vi "ASI_bufferToImage_Array.vi"(0 "iWidth":i32, 5 "iHeight":i32, 9 "imageType":i32, 11 "pBuffer in":u8[](array[numeric])) -> (10 "output array":u32[][](array[numeric]))   [LabVIEW 2023]
panel:
  in  "16bit type 2":u16[](array[numeric])
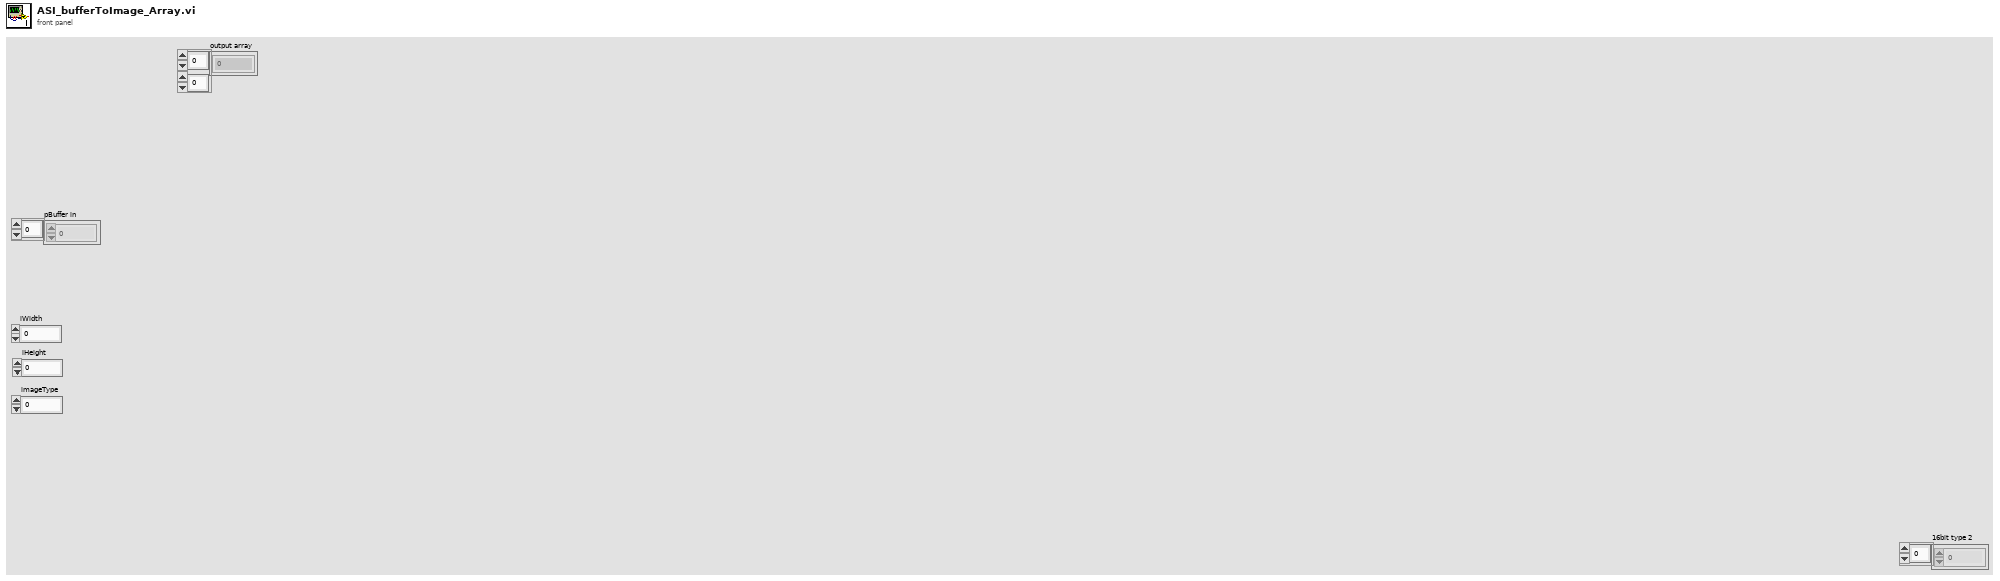
[diagram p1: front panel]
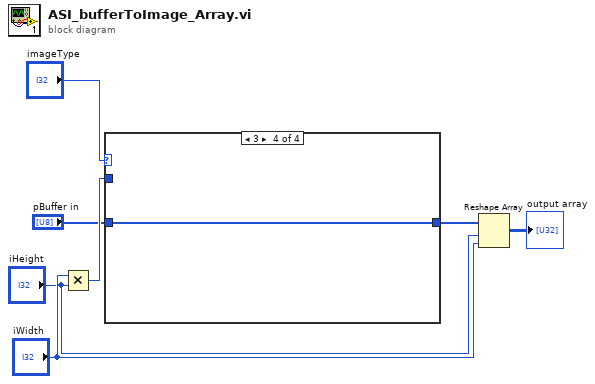
[diagram p0: block diagram]
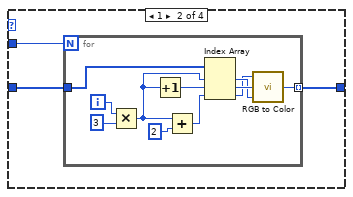
[diagram p3: hidden frame]
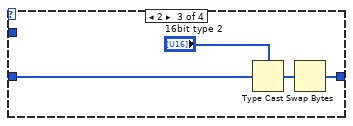
[diagram p4: hidden frame]
diagram:
  n1 = Multiply(x="iWidth", y="iHeight") -> (x*y=w7:i32)
  n2 = case shown="3" "imageType" {
    tunnel: [w8 w9 w23 w27] -> w6
    tunnel: "pBuffer in" -> [w8 w10 w24 w27]
    tunnel: w7 -> [_ w11 _ _]
    frame 0, Default {
    }
    frame 1 {
      n3 = for {
        N: w11 -> [_]
        tunnel: w10 -> [w21]
        tunnel: [w16] -> w9 mode=indexing
        i -> [w14]
        n4 = Multiply(x=w14, y=u16 3) -> (x*y=w15:i32)
        n5 = Increment(x=w15) -> (x+1=w20:i32)
        n6 = Add(x=w15, y=2 ("x")) -> (x+y=w19:i32)
        n7 = Index Array(array=w21, index #1=w15, index #2=w20, index #3=w19) -> (element #1=w13:u8, element #2=w17:u8, element #3=w12:u8)
        n8 = call <vilib>:"RGB to Color.vi"("B"=w13, "G"=w17, "R"=w12) -> ("Color"=w16:u32)
      }
    }
    frame 2 {
      n9 = Type Cast(type="16bit type 2", x=w24) -> (*(type *) &x=w25:u16[])
      n10 = Swap Bytes(anything=w25) -> (byte swapped=w23:u16[])
    }
    frame 3 {
    }
  }
  n11 = Reshape Array(w6, "iHeight", "iWidth") -> (→"output array":u32[][])
